vi "VISA update settings.vi"(8 "error in (no error)":errorcluster, 11 "AOTF in":refnum<class "Invivo_AOTF.lvclass">) -> (0 "error out":errorcluster, 3 "AOTF out":refnum<class "Invivo_AOTF.lvclass">)   [LabVIEW 2012, in "Invivo_AOTF.lvclass"]
uses:
  Invivo_AOTF.lvclass
  Invivo_AOTF.lvclass/Invivo_AOTF.ctl
panel:
  out "concatenated string":string
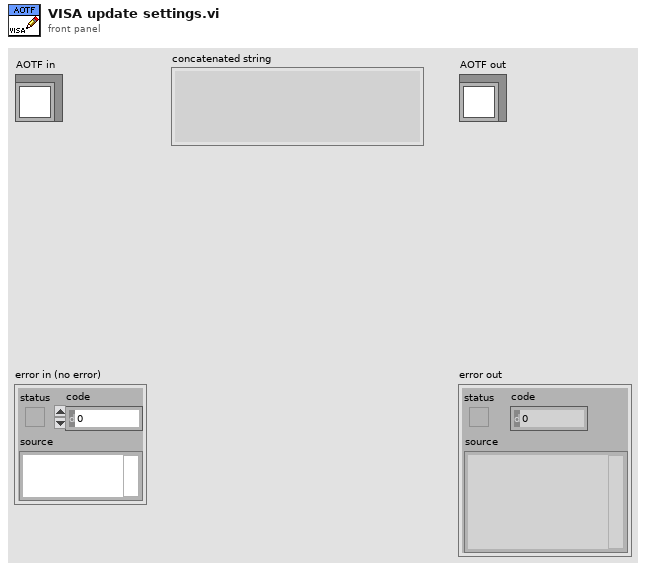
[diagram p1: front panel]
types:
  T1 = typedef "In vivo_AOTF.lvclass/laser line enum.ctl" = dbl
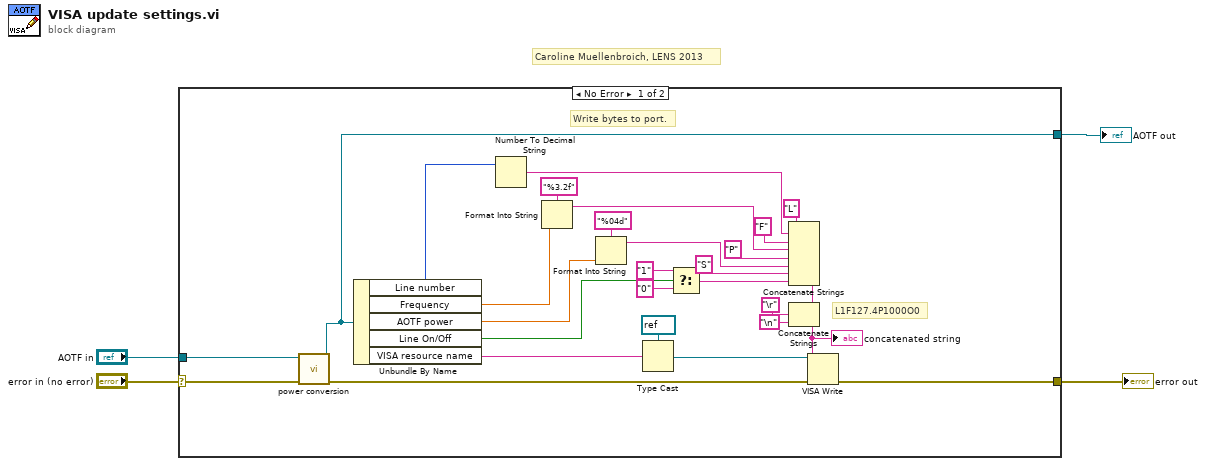
[diagram p0: block diagram]
diagram:
  # "Caroline Muellenbroich, LENS 2013"
  n1 = case shown="No Error" "error in (no error)" {
    selector: "error in (no error)" -> [w31 w34]
    tunnel: [w32 w34] -> w1
    tunnel: [w29 w33] -> w2
    tunnel: "AOTF in" -> [w30 w33]
    frame No Error {
      # "L1F127.4P1000O0"
      # "Write bytes to port."
      n2 = call-dynamic "power conversion.vi"("error in (no error)"=w31, "AOTF in"=w30) -> ("error out"=w5:errorcluster, "AOTF out"=w29:refnum<class "Invivo_AOTF.lvclass">)  [unwired: 8 in]
      n3 = Unbundle By Name(w29) -> ("Line number"=w17:u32, "Frequency"=w15:T1, "AOTF power"=w12:dbl, "Line On/Off"=w6:bool, "VISA resource name"=w20:string)
      n4 = Number To Decimal String(number=w17) -> (decimal integer string=w18:string)  [unwired: 1 in]
      n5 = Format Into String(format string="%3.2f", w15) -> (resulting string=w13:string)  [unwired: 2 in, 1 out]
      n6 = Format Into String(format string="%04d", w12) -> (resulting string=w11:string)  [unwired: 2 in, 1 out]
      n7 = Type Cast(type=refnum<visa-resource-name> refnum ("VISA resource name"), x=w20) -> (*(type *) &x=w16:refnum<visa-resource-name>)
      n8 = Select(t="1" ("string"), s=w6, f="0" ("string")) -> (s? t:f=w9:string)
      n9 = Concatenate Strings("L", w18, "F" ("string"), w13, "P" ("string"), w11, "S" ("string"), w9) -> (w28:string)
      n10 = Concatenate Strings(w28, "\r", "\n") -> (w22:string)
      "concatenated string" <- w22
      n11 = VISA Write(VISA resource name=w16, write buffer=w22, error in (no error)=w5) -> (error out=w32:errorcluster)  [unwired: 2 out]
    }
    frame Error {
    }
  }
  "error out" <- w1
  "AOTF out" <- w2
